vi "Connect_SignatureIn_QtSlot.vi"(4 "Slot Signature":string, 6 "Receiver":refnum<class "LQObject.lvclass">, 8 "Error In":errorcluster, 10 "Signal Signature":string, 11 "Sender In":refnum<class "LQObject.lvclass">) -> (0 "Error Out":errorcluster, 3 "Sender Out":refnum<class "LQObject.lvclass">)   [LabVIEW 2013, in "Template.lvlib" / "LQCoreEngine.lvclass"]
uses:
  LQCoreEngine.lvclass
  LQObject/LQObject.lvclass
  LQIdentity/LQIdentity.lvclass/LQIdentity.ctl
  LQIdentity/LQIdentity.lvclass
  Template.lvlib
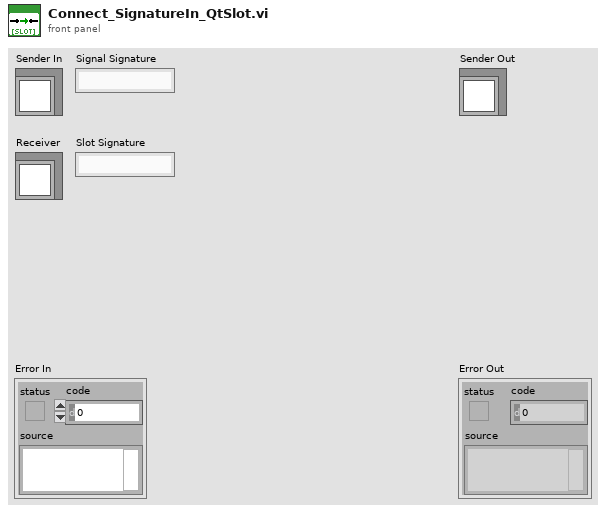
[diagram p1: front panel]
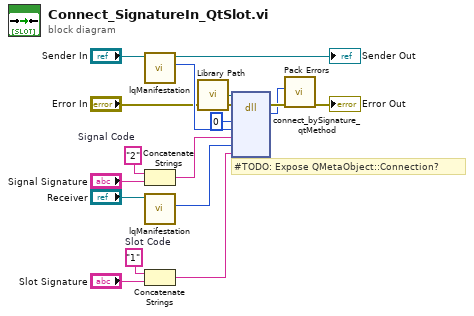
[diagram p0: block diagram]
diagram:
  w8 = "1"  # Slot Code
  w10 = "2"  # Signal Code
  # "#TODO: Expose QMetaObject::Connection?"
  n1 = call "lqManifestation.vi"("LQIdentity in"="Sender In") -> ("Manifestation"=w12:u64, "LQIdentity out"=→"Sender Out":refnum<class "LQObject.lvclass">)  [unwired: 9 in]
  n2 = Concatenate Strings(w10, "Signal Signature") -> (w5:string)
  n3 = call "lqManifestation.vi"("LQIdentity in"="Receiver") -> ("Manifestation"=w13:u64)  [unwired: 9 in, 1 out]
  n4 = Concatenate Strings(w8, "Slot Signature") -> (w6:string)
  n5 = call "Library Path.vi"() -> ("Library Path"=w16:path)
  n6 = dll-call lib="?" fn="connect_bySignature_qtMethod"(path in=w16, error in="Error In", "_retVal"=u64 0, "sender"=w12, "encodedSignal"=w5, "receiver"=w13, "encodedMethod"=w6) -> (error out=w4:errorcluster, "errorCode"=w3:i32)  [unwired: 6 in, 1 out]
  n7 = call "Pack Errors.vi"("Error In"=w4, "Error Code"=w3) -> ("Error Out"=→"Error Out":errorcluster)  [unwired: 9 in]
